vi "Yokogawa WT200 Series Measure Mode Value dryer.vi"(0 "VISA resource name":refnum<visa-resource-name>, 11 "error in (no error)":errorcluster) -> (8 "Measure Value":sgl[](array[numeric]) format="%^.3e", 15 "error out":errorcluster)   [LabVIEW 2016]
doc: "This VI configures measurement mode and measures voltage, current and active power for the element 1."
uses:
  Yokogawa WT200 Series.lvlib
panel:
  out "VISA resource name out":refnum<visa-resource-name>
  out "error message":string
  out "error":bool
  # "© 2005 National Instruments.  ALL RIGHTS RESERVED."
  # "WT200 SERIES"
  # "DIGITAL POWER METER"
  # "V1"
  # "v3"
  # "W(Sigma)"
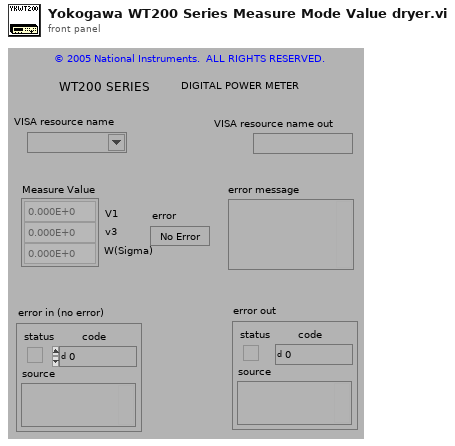
[diagram p1: front panel]
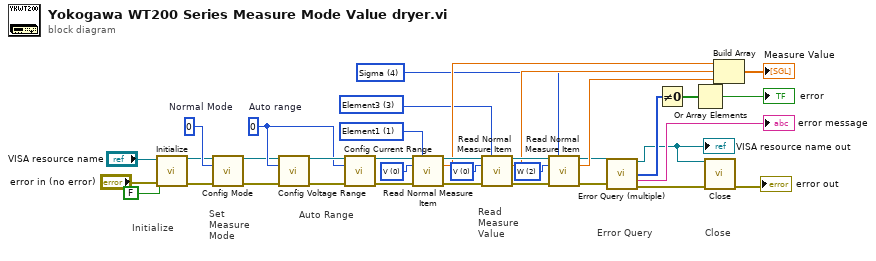
[diagram p0: block diagram]
diagram:
  w1 = u16 4 items=["", "Element1", "Element2", "Element3", "Sigma"] ("Element (1: Element 1)")
  w2 = u16 3 items=["", "Element1", "Element2", "Element3", "Sigma"] ("Element (1: Element 1)")
  w18 = u16 1 items=["", "Element1", "Element2", "Element3", "Sigma"] ("Element (1: Element 1)")
  w19 = u16 0 items=["V", "A", "W", "VA", "var", "PF", "deg", "V Hz", "A Hz", "Wh", "Wh+", "Wh-", "Ah", "Ah+", "Ah-", "Vpk", "Apk", "Math"] ("Measure Item (0: V)")
  w20 = u16 2 items=["V", "A", "W", "VA", "var", "PF", "deg", "V Hz", "A Hz", "Wh", "Wh+", "Wh-", "Ah", "Ah+", "Ah-", "Vpk", "Apk", "Math"] ("Measure Item (0: V)")
  w21 = u16 0 items=["V", "A", "W", "VA", "var", "PF", "deg", "V Hz", "A Hz", "Wh", "Wh+", "Wh-", "Ah", "Ah+", "Ah-", "Vpk", "Apk", "Math"] ("Measure Item (0: V)")
  w33 = u16 0  # Auto range
  w36 = u16 0  # Normal Mode
  # "Error Query"
  # "Close"
  # "Initialize"
  # "Read\nMeasure\nValue"
  # "Auto Range"
  # "Set \nMeasure \nMode"
  n1 = call "Initialize.vi"("VISA resource name"="VISA resource name", "Reset (T: Reset)"=FALSE, "error in (no error)"="error in (no error)") -> ("VISA resource name out"=w15:refnum<visa-resource-name>, "error out"=w14:errorcluster)  [unwired: 10 in, 1 out]
  n2 = call "Config Mode.vi"("VISA resource name"=w15, "Mode (0: RMS)"=w36, "error in (no error)"=w14) -> ("VISA resource name out"=w32:refnum<visa-resource-name>, "error out"=w31:errorcluster)  [unwired: 11 in]
  n3 = call "Config Voltage Range.vi"("VISA resource name"=w32, "V Range (6: 600V)"=w33, "error in (no error)"=w31) -> ("VISA resource name out"=w34:refnum<visa-resource-name>, "error out"=w35:errorcluster)  [unwired: 11 in]
  n4 = call "Config Current Range.vi"("VISA resource name"=w34, "A Range (12: 20A)"=w33, "error in (no error)"=w35) -> ("VISA resource name out"=w29:refnum<visa-resource-name>, "error out"=w30:errorcluster)  [unwired: 11 in]
  n5 = call "Read Normal Measure Item.vi"("VISA resource name"=w29, "Element (1: Element 1)"=w18, "Measure Item (0: V)"=w19, "error in (no error)"=w30) -> ("VISA resource name out"=w26:refnum<visa-resource-name>, "Measure Value"=w22:sgl, "error out"=w28:errorcluster)  [unwired: 9 in]
  n6 = call "Read Normal Measure Item.vi"("VISA resource name"=w26, "Element (1: Element 1)"=w2, "Measure Item (0: V)"=w21, "error in (no error)"=w28) -> ("VISA resource name out"=w25:refnum<visa-resource-name>, "Measure Value"=w23:sgl, "error out"=w27:errorcluster)  [unwired: 9 in]
  n7 = call "Read Normal Measure Item.vi"("VISA resource name"=w25, "Element (1: Element 1)"=w1, "Measure Item (0: V)"=w20, "error in (no error)"=w27) -> ("VISA resource name out"=w11:refnum<visa-resource-name>, "Measure Value"=w24:sgl, "error out"=w10:errorcluster)  [unwired: 9 in]
  n8 = call "Error Query (multiple).vi"("VISA resource name"=w11, "error in (no error)"=w10) -> ("VISA resource name out"=w4:refnum<visa-resource-name>, "Error"=w7:i32[], "Error Message"=→"error message":string, "error out"=w6:errorcluster)  [unwired: 10 in]
  "VISA resource name out" <- w4
  n9 = Not Equal To 0?(x=w7) -> (x != 0?=w8:bool[])
  n10 = Or Array Elements(Boolean array=w8) -> (logical OR=→"error":bool)
  n11 = call "Close.vi"("VISA resource name"=w4, "error in (no error)"=w6) -> ("error out"=→"error out":errorcluster)  [unwired: 13 in]
  n12 = Build Array(w22, w23, w24) -> (→"Measure Value":sgl[])
